vi "GPIB_autodetect.vi"(8 "error in (no error)":errorcluster, 9 "Verify GPIB address":bool, 10 "Instrument GPIB address in":string, 11 "KE487 in":refnum<class "KE487.lvclass">) -> (0 "error out":errorcluster, 2 "Instrument GPIB address":string, 3 "KE487 out":refnum<class "KE487.lvclass">)   [LabVIEW 2013, in "KE487.lvclass"]
uses:
  KE487.lvclass
  InstrControl.lvclass
panel:
  out "GPIB addresses found":string[](array[string])
  out "IDN? responses":string[](array[string])
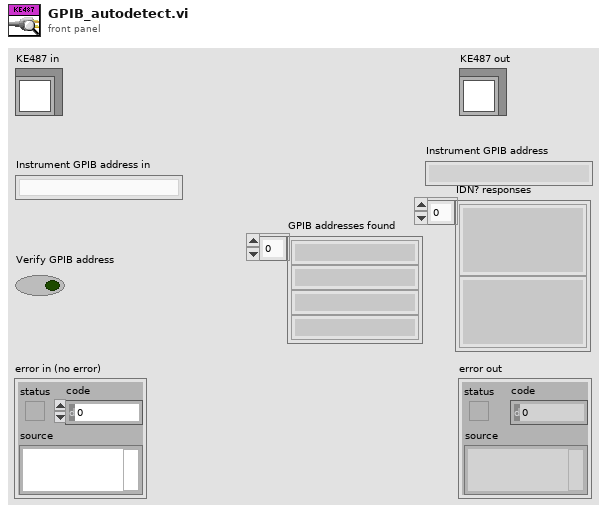
[diagram p1: front panel]
types:
  T1 = cluster{"error":bool, "code":i32, "source":string}
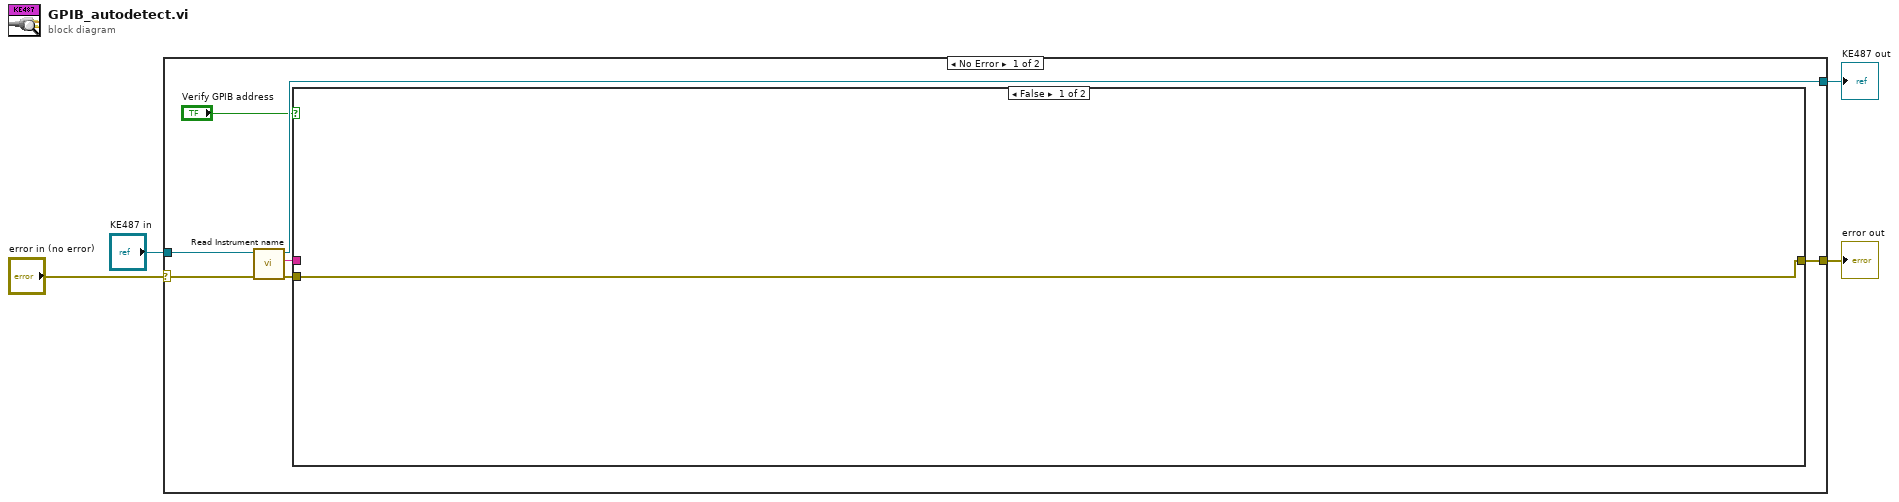
[diagram p0: block diagram]
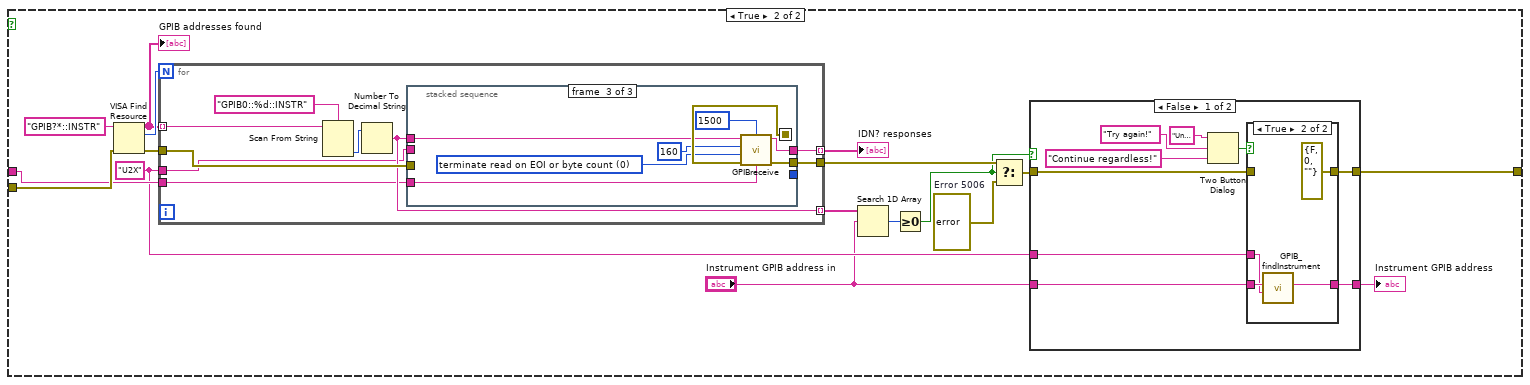
[diagram p2: hidden frame]
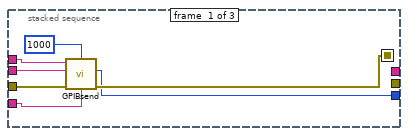
[diagram p5: hidden frame]
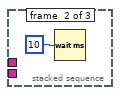
[diagram p6: hidden frame]
diagram:
  n1 = case shown="No Error" "error in (no error)" {
    selector: "error in (no error)" -> [w10 w73]
    tunnel: [w7 w73] -> w1
    tunnel: [w9 w72] -> w4
    tunnel: "KE487 in" -> [w11 w72]
    frame No Error {
      n2 = call-dynamic "Read Instrument name.vi"("error in (no error)"=w10, "InstControl in"=w11) -> ("error out"=w8:errorcluster, "Instrument name"=w6:string, "InstControl out"=w9:refnum<class "KE487.lvclass">)  [unwired: 7 in]
      n3 = case shown="False" "Verify GPIB address" {
        tunnel: w8 -> [w12 w23]
        tunnel: [w12 w17] -> w7
        tunnel: w6 -> [_ w16]
        frame False {
        }
        frame True {
          w14 = "U2X"
          w28 = errorcluster {"status"=FALSE, "code"=5005, "source"="Unable to find specified instrument.  Please make sure the it is connected to your system and switched on."}  # Error 5006
          n4 = VISA Find Resource(8:w23, 11:"GPIB?*::INSTR" ("expression (\"\")")) -> (0:w27:errorcluster, 2:w26:u32, 3:w25:string[])  [unwired: 1 in]
          "GPIB addresses found" <- w25
          n5 = for {
            N: w26 -> [_]
            tunnel: w25 -> [w53] mode=indexing
            tunnel: w27 -> [w55]
            tunnel: [w54] -> w29
            tunnel: [w49] -> w21 mode=indexing
            tunnel: w16 -> [w48]
            tunnel: [w50] -> w24 mode=indexing
            tunnel: w14 -> [w47]
            n6 = Scan From String(format string="GPIB0::%d::INSTR" ("expression (\"\")"), input string=w53) -> (output 1=w51:i32)  [unwired: 3 in, 3 out]
            n7 = Number To Decimal String(number=w51) -> (decimal integer string=w49:string)  [unwired: 1 in]
            n8 = stacked-sequence {
              seq-local: [w60 _ _] -> [_ _ w70]
              tunnel: w49 -> [w62 _ w69]
              tunnel: w55 -> [w61 _ _]
              tunnel: [_ _ w71] -> w54
              tunnel: [_ _ w66] -> w50
              tunnel: w48 -> [w58 _ w67]
              tunnel: w47 -> [w57 _ _]
              tunnel: [w56 _ _] -> _
              frame #0 {
                n9 = call "GPIBsend.vi"("timeout ms"=u32 1000, "address string"=w62, "write buffer"=w57, "source"=w58, "error in"=w61) -> ("byte count"=w56:i32, "error out"=w60:errorcluster)  [unwired: 2 in, 1 out]
              }
              frame #1 {
                n10 = Wait (ms)(milliseconds to wait=10) -> ()  [unwired: 1 out]
              }
              frame #2 {
                w65 = 0 items=["terminate read on EOI or byte count", "terminate read on EOI, byte count, or CR", "terminate read on EOI, byte count, or LF"] ("read mode")
                n11 = call "GPIBreceive.vi"("timeout ms"=u32 1500, "address string"=w69, "byte count"=160, "source"=w67, "read mode"=w65, "error in"=w70) -> ("read buffer"=w66:string, "error out"=w71:T1)  [unwired: 1 in, 1 out]
              }
            }
          }
          "IDN? responses" <- w24
          n12 = Search 1D Array(1D array=w21, element="Instrument GPIB address in") -> (index of element=w20:i32)  [unwired: 1 in]
          n13 = Greater Or Equal To 0?(x=w20) -> (x >= 0?=w19:bool)
          n14 = Select(t=w29, s=w19, f=w28) -> (s? t:f=w18:errorcluster)
          n15 = case shown="False" w19 {
            tunnel: "Instrument GPIB address in" -> [w34 w46]
            tunnel: [w33 w46] -> w15
            tunnel: w18 -> [w32 w45]
            tunnel: [w31 w45] -> w17
            tunnel: w14 -> [w30 _]
            frame False {
              n16 = Two Button Dialog(message="Unable to find specified instrument.  Please make sure the it is connected to your system and switched on." ("source"), 1:"Continue regardless!", 2:"Try again!") -> (T button?=w35:bool)
              n17 = case shown="True" w35 {
                tunnel: w34 -> [w40 w44]
                tunnel: [w40 w43] -> w33
                tunnel: w32 -> [w39 _]
                tunnel: [w39 errorcluster {"status"=FALSE, "code"=0, "source"=""} ("error constant")] -> w31
                tunnel: w30 -> [_ w41]
                frame False {
                }
                frame True {
                  n18 = call "GPIB_findInstrument.vi"("ID command"=w41, "revised GPIB address"=w44) -> ("revised GPIB address OUT"=w43:string)  [unwired: 9 in]
                }
              }
            }
            frame True {
            }
          }
          "Instrument GPIB address" <- w15
        }
      }
    }
    frame Error {
    }
  }
  "error out" <- w1
  "KE487 out" <- w4
